vi "Build.vi"(8 "error in (no error)":errorcluster, 11 "Project Builder in":refnum<class "Project Builder.lvclass">) -> (0 "error out":errorcluster, 1 "Success?":bool, 3 "Project Builder out":refnum<class "Project Builder.lvclass">)   [LabVIEW 2019, in "ProjectBuilder.lvlib" / "Project Builder.lvclass"]
doc: "Load and execute all actions."
uses:
  Project Builder.lvclass
  Project Builder.lvclass/Project Builder.ctl
  Ctl/Ctl_Build Steps.ctl
  Report Action/Report Action/Report Action.lvclass
  C:/WS/prev/LV32.2019..ProjectBuilder/Class/Project Action/Project Action.lvclass
  <vilib>/Utility/error.llb/Error Cluster From Error Code.vi
  <vilib>/ErrorRing/Error Ring.xnode
  ProjectBuilder.lvlib
  <vilib>/Utility/Data Type/NI_Data Type.lvlib
  PPL/HDH.ClassLoader.lvlibp
  Project Action/Project Action.lvclass
panel:
  out "Active Action":string
  out "Sub-Progress":i32(slide) caption="Progress: Sub" scale=0.0..10.0
  out "Progress: Total":i32(slide) scale=0.0..10.0
  out "Active Project":path
  in  "Abort":bool
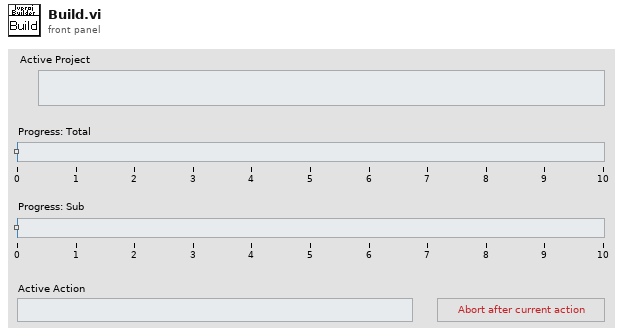
[diagram p1: front panel]
types:
  T1 = typedef "ProjectBuilder.lvlib/Ctl_Build Steps.ctl" = enum16{"Source Test", "Build", "Post-Build Test", "Deploy", "Report"}
  T2 = typedef "ProjectBuilder.lvlib/Project Builder.lvclass/Ctl_Run Cluster.ctl" = cluster{"Source Tests":refnum<class "Project Action.lvclass">[], "Build Array":refnum<class "Project Action.lvclass">[], "Post-Build Tests":refnum<class "Project Action.lvclass">[], "Deploy Array":refnum<class "Project Action.lvclass">[], "Report Handler Array":refnum<class "Report Action.lvclass">[], "Element Count":i32}
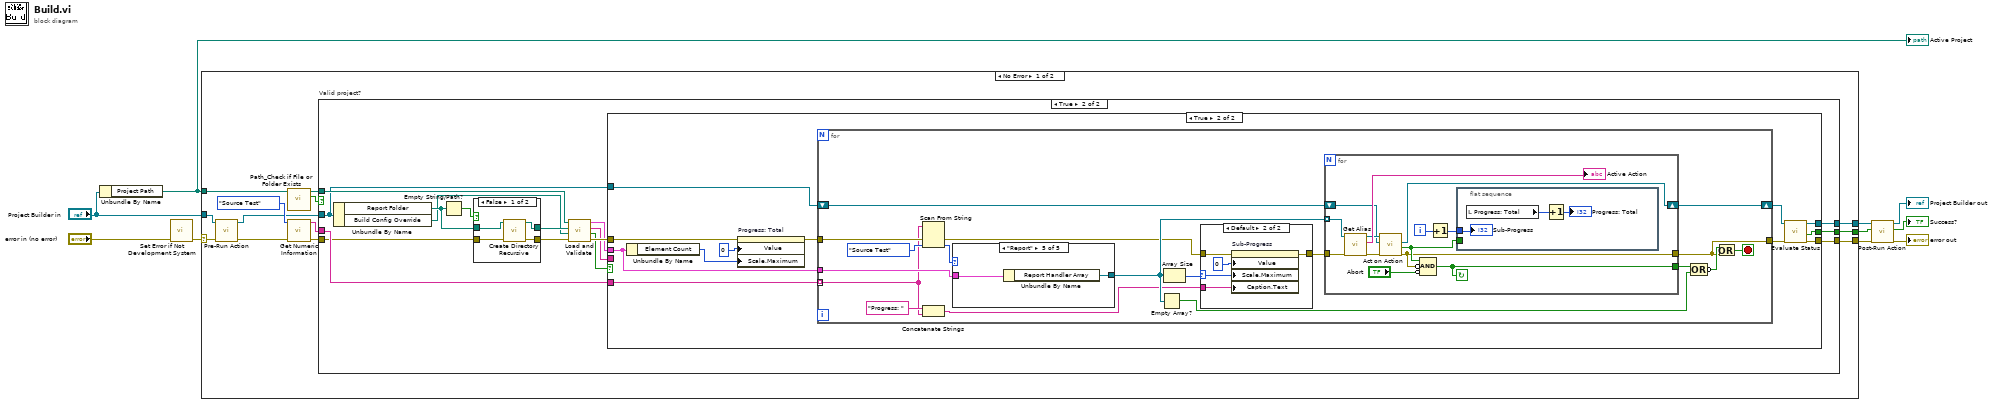
[diagram p0: block diagram]
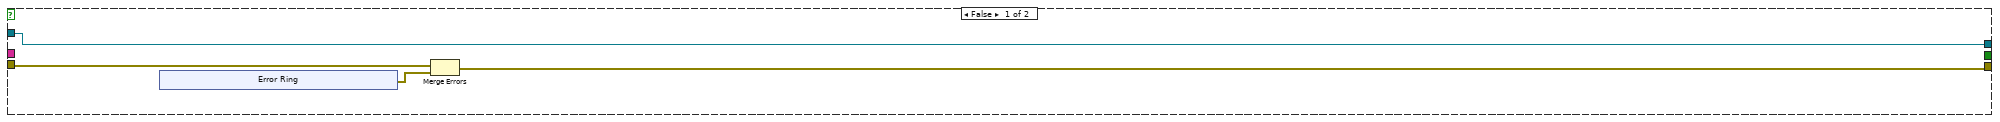
[diagram p2: hidden frame]
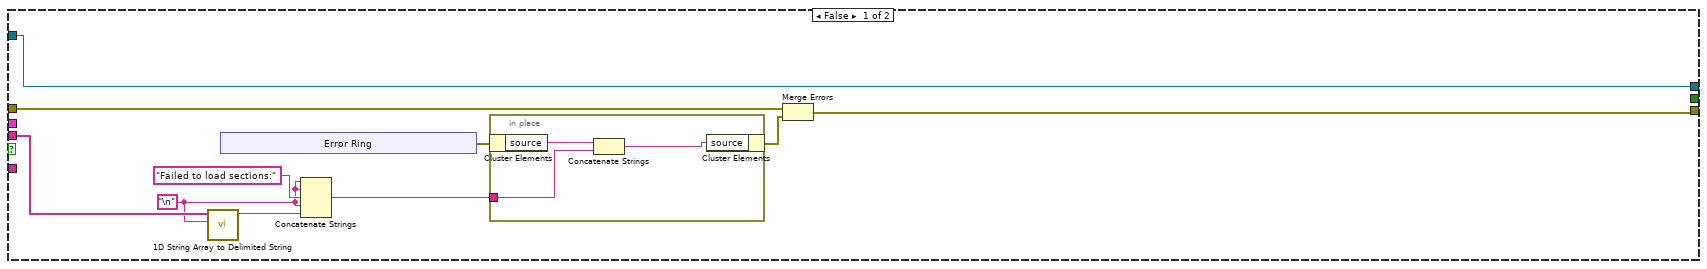
[diagram p4: hidden frame]
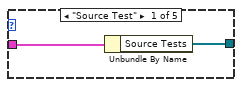
[diagram p6: hidden frame]
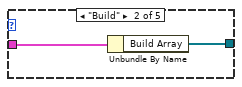
[diagram p7: hidden frame]
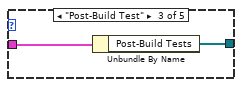
[diagram p8: hidden frame]
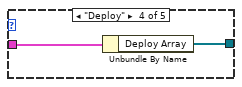
[diagram p9: hidden frame]
diagram:
  n1 = Unbundle By Name("Project Builder in") -> ("Project Path"=w6:path)
  "Active Project" <- w6
  n2 = call "Set Error if Not Development System.vi"("error in (no error)"="error in (no error)") -> ("error out"=w8:errorcluster)  [unwired: 10 in]
  n3 = case shown="No Error" w8 {
    selector: w8 -> [w22 w134]
    tunnel: w6 -> [w23 _]
    tunnel: [w19 w134] -> w10
    tunnel: [w18 _] -> w2
    tunnel: [w14 w133] -> w4
    tunnel: "Project Builder in" -> [w12 w133]
    frame No Error {
      n4 = call-dynamic "Pre-Run Action.vi"("error in (no error)"=w22, "Project Builder in"=w12) -> ("error out"=w13:errorcluster, "Project Builder out"=w11:refnum<class "Project Builder.lvclass">)  [unwired: 8 in]
      n5 = call "Path_Check if File or Folder Exists.vi"("File or Folder Path in"=w23) -> ("File or Folder Found?"=w21:bool, "File or Folder Path dub"=w20:path)  [unwired: 9 in]
      n6 = call <vilib>:"Get Numeric Information.vi"("error in (no error)"=w13, "variant"=Ctl_Build_Steps."Source Test" ("Build Step")) -> ("error out"=w15:errorcluster, "enum names"=w17:string[])  [unwired: 6 in, 2 out]
      n7 = case "Valid project?" shown="True" w21 {
        tunnel: [w25 w47] -> w19
        tunnel: w15 -> [w27 w35]
        tunnel: w20 -> [_ w46]
        tunnel: [_ w41] -> w18
        tunnel: w17 -> [_ w40]
        tunnel: w11 -> [w24 w38]
        tunnel: [w24 w39] -> w14
        frame False {
          n8 = xnode "Error Ring"() -> ("error out"=w26:errorcluster)
          n9 = Merge Errors(w27, w26) -> (w25:errorcluster)
        }
        frame True {
          n10 = Unbundle By Name(w38) -> ("Report Folder"=w33:path, "Build Config Override"=w32:path)
          n11 = Empty String/Path?(string/path=w33) -> (empty?=w37:bool)
          n12 = case shown="False" w37 {
            tunnel: [w48 w53] -> w36
            tunnel: w35 -> [w51 w53]
            tunnel: [w49 w52] -> w34
            tunnel: w33 -> [w50 w52]
            frame False {
              n13 = call <vilib>:"Create Directory Recursive.vi"("error in (no error)"=w51, "directory"=w50) -> ("error out"=w48:errorcluster, "directory copy"=w49:path)  [unwired: 3 in, 1 out]
            }
            frame True {
            }
          }
          n14 = call "Load and Validate.vi"("error in (no error)"=w36, "Build Config Override"=w32, "Report Folder"=w34, "Project Path"=w46) -> ("error out"=w45:errorcluster, "Valid?"=w43:bool, "Invalid Sections"=w42:string[], "Run cluster"=w44:T2)  [unwired: 4 in]
          n15 = case shown="True" w43 {
            tunnel: [w62 w72] -> w47
            tunnel: w45 -> [w63 w78]
            tunnel: w44 -> [_ w81]
            tunnel: w42 -> [w59 _]
            tunnel: [_ w71] -> w41
            tunnel: w40 -> [_ w82]
            tunnel: [w54 w74] -> w39
            tunnel: w38 -> [w54 w76]
            frame False {
              w55 = "\n"
              n16 = call <vilib>:"1D String Array to Delimited String.vi"("delimiter"=w55, "string array"=w59) -> ("delimited string"=w57:string)  [unwired: 9 in]
              n17 = xnode "Error Ring"() -> ("error out"=w61:errorcluster)
              n18 = Concatenate Strings(w55, w55, "Failed to load sections:", w55, w57) -> (w56:string)
              n19 = in-place {
                in-place-border: w56 -> [w65]
                n20 = in-place-cluster #1(w61) -> ("source"=w66:string)
                n21 = Concatenate Strings(w66, w65) -> (w64:string)
                n22 = in-place-cluster #1("source"=w64) -> (w60:errorcluster)
              }
              n23 = Merge Errors(w63, w60) -> (w62:errorcluster)
            }
            frame True {
              n24 = Unbundle By Name(w81) -> ("Element Count"=w80:i32)
              n25 = property on="Progress: Total" class="Slide (strict)"(error in=w78, "Value"=0 ("Progress: Total"), "Scale.Maximum"=w80) -> (error out=w77:errorcluster)  [unwired: 1 in, 1 out]
              n26 = for {
                tunnel: w77 -> [w93]
                tunnel: [w95] -> w73
                tunnel: w81 -> [w100]
                tunnel: w82 -> [w87] mode=indexing
                shift-right: [w84] -> w75
                shift-left: w76 -> [w85]
                stop <- w97 stop-if-true
                n27 = Scan From String(input string=w87, error in=w93, default 1=Ctl_Build_Steps."Source Test" ("Build Step")) -> (error out=w83:errorcluster, output 1=w92:T1)  [unwired: 2 in, 2 out]
                n28 = Concatenate Strings("Progress: " ("string"), w87) -> (w86:string)
                n29 = case shown="\"Report\"" w92 {
                  tunnel: w100 -> [w124 w126 w128 w130 w132]
                  tunnel: [w123 w125 w127 w129 w131] -> w91
                  frame "Source Test" {
                    n30 = Unbundle By Name(w124) -> ("Source Tests"=w123:refnum<class "Project Action.lvclass">[])
                  }
                  frame "Build" {
                    n31 = Unbundle By Name(w126) -> ("Build Array"=w125:refnum<class "Project Action.lvclass">[])
                  }
                  frame "Post-Build Test" {
                    n32 = Unbundle By Name(w128) -> ("Post-Build Tests"=w127:refnum<class "Project Action.lvclass">[])
                  }
                  frame "Deploy" {
                    n33 = Unbundle By Name(w130) -> ("Deploy Array"=w129:refnum<class "Project Action.lvclass">[])
                  }
                  frame "Report" {
                    n34 = Unbundle By Name(w132) -> ("Report Handler Array"=w131:refnum<class "Report Action.lvclass">[])
                  }
                }
                n35 = Empty Array?(array=w91) -> (empty?=w96:bool)
                n36 = Array Size(array=w91) -> (size(s)=w90:i32)
                n37 = case shown="Default" w90 {
                  selector: w90 -> [_ w105]
                  tunnel: w83 -> [w101 w104]
                  tunnel: [w101 w103] -> w89
                  tunnel: w86 -> [_ w102]
                  frame 0 {
                  }
                  frame Default {
                    n38 = property on="Sub-Progress" class="Slide (strict)"(error in=w104, "Value"=0 ("Progress: Total"), "Scale.Maximum"=w105, "Caption.Text"=w102) -> (error out=w103:errorcluster)  [unwired: 1 in, 1 out]
                  }
                }
                n39 = for {
                  tunnel: w91 -> [w114] mode=indexing
                  tunnel: w89 -> [w119]
                  tunnel: [w107] -> w95
                  tunnel: [w118] -> w99
                  shift-right: [w110] -> w84
                  shift-left: w85 -> [w111]
                  i -> [w116]
                  stop <- w118 continue-if-true
                  n40 = call "Get Alias.vi"("error in (no error)"=w119, "Project Action in"=w114) -> ("error out"=w109:errorcluster, "Alias"=→"Active Action":string, "Project Action out"=w112:refnum<class "Project Action.lvclass">)  [unwired: 7 in]
                  n41 = call "Act on Action.vi"("error in (no error)"=w109, "Project Builder in"=w111, "Project Action in"=w112) -> ("error out"=w107:errorcluster, "Continue?"=w108:bool, "Project Builder out"=w110:refnum<class "Project Builder.lvclass">)  [unwired: 6 in]
                  n42 = Compound Arithmetic op=AND(w108, invert w107, invert "Abort") -> (w118:bool)
                  n43 = Increment(x=w116) -> (x+1=w115:i32)
                  n44 = flat-sequence {
                    tunnel: w115 -> [w122]
                    tunnel: w108 -> [_]
                    frame #0 {
                      n45 = local read "Progress: Total"() -> (w120:i32)
                      n46 = Increment(x=w120) -> (x+1=→"Progress: Total":i32)
                      "Sub-Progress" <- w122
                    }
                  }
                }
                n47 = Compound Arithmetic op=OR(w99, w96) -> (invert w98:bool)
                n48 = Or(x=w98, y=w95) -> (x .or. y?=w97:bool)
              }
              n49 = call "Evaluate Status.vi"("error in (no error)"=w73, "Project Builder in"=w75) -> ("error out"=w72:errorcluster, "Passed?"=w71:bool, "Project Builder out"=w74:refnum<class "Project Builder.lvclass">)  [unwired: 7 in]
            }
          }
        }
      }
    }
    frame Error {
    }
  }
  n50 = call-dynamic "Post-Run Action.vi"("error in (no error)"=w10, "Passed? in"=w2, "Project Builder in"=w4) -> ("error out"=→"error out":errorcluster, "Passed? out"=→"Success?":bool, "Project Builder out"=→"Project Builder out":refnum<class "Project Builder.lvclass">)  [unwired: 6 in]
